vi "IV_Model.vi"(3 "output control":T1, 4 "data":variant, 5 "X":dbl[](array[numeric]), 6 "a":dbl[](array[numeric])) -> (0 "error out":errorcluster, 1 "f'(X,a)":dbl[][](array[numeric]), 2 "f(X,a)":dbl[](array[numeric]))   [LabVIEW 2020]
doc: "Implements an ellipse model function to be passed to the Nonlinear Curve Fit.vi."
uses:
  <vilib>/gmath/NumericalOptimization/LM_output select.ctl
  <vilib>/gmath/NI_Gmath.lvlib
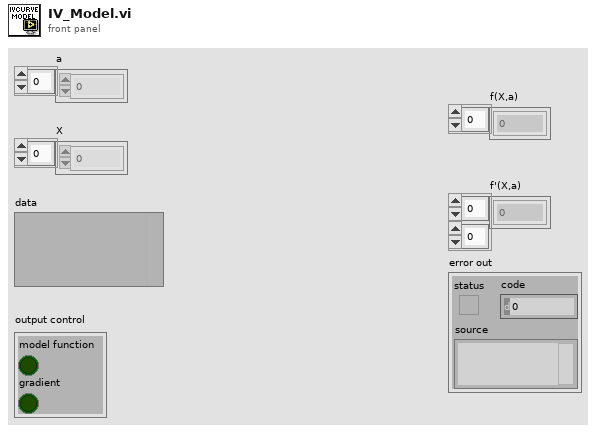
[diagram p1: front panel]
types:
  T1 = typedef "NI_Gmath.lvlib/LM_output select.ctl" = cluster{"model function":bool, "gradient":bool}
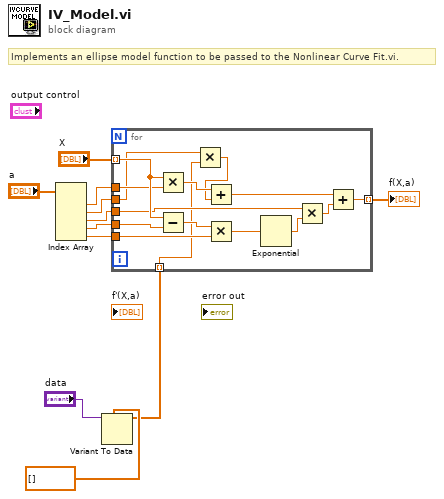
[diagram p0: block diagram]
diagram:
  # "Implements an ellipse model function to be passed to the Nonlinear Curve Fit.vi."
  n1 = Index Array(array="a") -> (element #1=w8:dbl, element #2=w7:dbl, element #3=w6:dbl, element #4=w5:dbl, element #5=w4:dbl)  [unwired: 5 in]
  n2 = Variant To Data(type=dbl[] [] ("a"), Variant="data") -> (data=w1:dbl[])  [unwired: 1 in, 1 out]
  n3 = for {
    tunnel: [w19] -> w11 mode=indexing
    tunnel: "X" -> [w24] mode=indexing
    tunnel: w8 -> [w18]
    tunnel: w7 -> [w12]
    tunnel: w6 -> [w17]
    tunnel: w5 -> [w16]
    tunnel: w4 -> [w15]
    tunnel: w1 -> [w13] mode=indexing
    n4 = Multiply(x=w24, y=w18) -> (x*y=w26:dbl)
    n5 = Subtract(x=w24, y=w16) -> (x-y=w23:dbl)
    n6 = Multiply(x=w12, y=w13) -> (x*y=w14:dbl)
    n7 = Add(x=w26, y=w14) -> (x+y=w21:dbl)
    n8 = Multiply(x=w23, y=w15) -> (x*y=w22:dbl)
    n9 = Exponential(1:w22) -> (0:w25:dbl)
    n10 = Multiply(x=w17, y=w25) -> (x*y=w20:dbl)
    n11 = Add(x=w21, y=w20) -> (x+y=w19:dbl)
  }
  "f(X,a)" <- w11
